vi "Display name.vi"(1 "State In":T1) -> (0 "Name":string)   [LabVIEW 2018, in "OpenG FilterArray.xnode"]
uses:
  OpenG FilterArray.xnode
  State.ctl
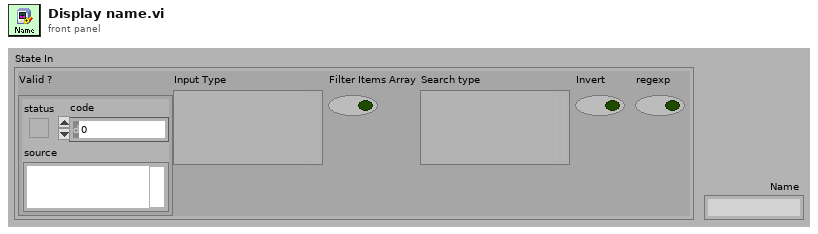
[diagram p1: front panel]
types:
  T1 = typedef "OpenG FilterArray.xnode/State.ctl" = cluster{"Valid ?":errorcluster, "Input Type":variant, "Filter Items Array":bool, "Search type":variant, "Invert":bool, "regexp":bool}
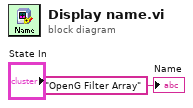
[diagram p0: block diagram]
diagram:
  "Name" <- "OpenG Filter Array" ("Name")
